vi "STS at various H_MFLI_MF-MD_K3636B_PK_V4.0_withaveraging.vi"() -> ()   [LabVIEW 2016]
uses:
  <instrlib>/Zurich Instruments LabOne/Public/Data/ziTypeDemodSampleSingle.ctl
  <instrlib>/Keithley 2600 Series/Public/Configure/Source/Configure Source (Limit).vi
  <instrlib>/Keithley 2600 Series/Public/Configure/Source/Configure Source (Range).vi
  <instrlib>/Zurich Instruments LabOne/Public/Configure/ziGetValueDemodSampleEx.vi
  <instrlib>/Zurich Instruments LabOne/Zurich Instruments LabOne.lvlib
  <instrlib>/Keithley 2600 Series/Keithley 2600 Series.lvlib
panel:
  in  "DC Current Limit (A)":dbl format="%#_13g"
  in  "Keithley 2636B (channelA)":refnum<visa-resource-name>
  in  "Field ramp rate (T/min)":string="0.05"
  in  "Step 2":dbl[](array[numeric])=[0.005] min=-3000.0 max=3000.0 format="%.1e"
  in  "To 2":dbl[](array[numeric])=[-5.0] min=-3000.0 max=3000.0 format="%.1e"
  in  "From 2":dbl[](array[numeric])=[5.0] min=-3000.0 max=3000.0 format="%.1e"
  in  "Magnet IP Address":string="169.254.46.132"
  in  "Magnetic field stabilization time (s)":dbl=200.0 format="%#_13g"
  out "Magnetic Field (T)":dbl format="%#_13g"
  in  "DC Voltage averaging":dbl=10.0 format="%#_13g"
  out "Demod Sample Out 2":T1={"Timestamps (ticks)"=34359738372, "X (Vrms)"=8.366245757779461e-285, "Y (Vrms)"=1.0096057436928657e-284, "Osc Phase (deg)"=1.69759663376e-313, "Freq (Hz)"=2.607691286315397e-191, "DIO"=4, "AuxIn0 (V)"=0.0, "AuxIn1 (V)"=1.6954746369817e-311, "Trigger"=16}
  out "Demod Sample Out":T1={"Timestamps (ticks)"=34359738372, "X (Vrms)"=8.366245757779461e-285, "Y (Vrms)"=1.0096057436928657e-284, "Osc Phase (deg)"=1.69759663376e-313, "Freq (Hz)"=2.607691286315397e-191, "DIO"=4, "AuxIn0 (V)"=0.0, "AuxIn1 (V)"=1.6954746369817e-311, "Trigger"=16}
  out "Vset (V)":dbl
  in  "stop":bool
  out "Time(s)":dbl
  in  "Delay (s)":dbl=12.0
  out "dI/dV (S)":dbl
  out "dV (V)":dbl
  out "dI (A)":dbl
  in  "MFLI Address":string="DEV4382"
  out "DC Voltage (V)":dbl
  in  "Folder":path=path "D:/Yaojia/KV3Sb5_JJ_004/21-05-2020"
  out "dI/dV vs Voltage":cluster{dbl, "Field Reading":dbl}[](graph)=[{0.0, "Field Reading"=0.0}, {0.0293132694, "Field Reading"=0.0001}, {-0.00546459921, "Field Reading"=0.0002}, {0.0161308434, "Field Reading"=0.00030000000000000003}, {0.0223832692, "Field Reading"=0.0004}, {0.0328436404, "Field Reading"=0.0005}, {0.038420414, "Field Reading"=0.0006000000000000001}, {0.0417674657, "Field Reading"=0.0007000000000000001}, {0.0438858754, "Field Reading"=0.0008000000000000001}, {0.0446854721, "Field Reading"=0.0009000000000000002}, {0.044680018, "Field Reading"=0.001}, {0.0438771516, "Field Reading"=0.0009}, {0.0430695093, "Field Reading"=0.0007999999999999999}, {0.0423949057, "Field Reading"=0.0006999999999999999}, {0.0424006302, "Field Reading"=0.0005999999999999998}, {0.0430089846, "Field Reading"=0.0004999999999999998}, {0.0431435269, "Field Reading"=0.0003999999999999998}, {0.0431290947, "Field Reading"=0.0002999999999999998}, {0.0703335255, "Field Reading"=0.00019999999999999982}, {0.0575145557, "Field Reading"=9.999999999999982e-05}, {0.11367481, "Field Reading"=-1.8973538018496328e-19}, {0.109008679, "Field Reading"=-0.0001000000000000002}, {0.0119374597, "Field Reading"=-0.0002000000000000002}, {-0.0231964252, "Field Reading"=-0.0003000000000000002}, {-0.0302370322, "Field Reading"=-0.0004000000000000002}, {-0.0435009579, "Field Reading"=-0.0005000000000000002}, {-0.0500857587, "Field Reading"=-0.0006000000000000003}, {-0.0527825661, "Field Reading"=-0.0007000000000000003}, {-0.0535569139, "Field Reading"=-0.0008000000000000004}, {-0.0533778669, "Field Reading"=-0.0009000000000000004}, {-0.0526966423, "Field Reading"=-0.001}, {-0.0518844802, "Field Reading"=-0.0009}, {-0.051037725, "Field Reading"=-0.0007999999999999999}, {-0.0502346264, "Field Reading"=-0.0006999999999999999}, {-0.0495006625, "Field Reading"=-0.0005999999999999998}, {-0.0488631228, "Field Reading"=-0.0004999999999999998}, {-0.0482498135, "Field Reading"=-0.0003999999999999998}, {-0.0476401668, "Field Reading"=-0.0002999999999999998}, {-0.0812013466, "Field Reading"=-0.00019999999999999982}, {-0.0619737297, "Field Reading"=-9.999999999999982e-05}]
  out "data":dbl[](array[numeric])=[-0.0619737297, -9.999999999999982e-05, 619.7372970000011]
  in  "Nanovoltmeter 2182a VISA":refnum<visa-resource-name>="GPIB0::7::INSTR"
  in  "Step":dbl[](array[numeric])=[0.005] min=-3000.0 max=3000.0 format="%.1e"
  in  "To":dbl[](array[numeric])=[-5.0] min=-3000.0 max=3000.0 format="%.1e"
  in  "From":dbl[](array[numeric])=[5.0] min=-3000.0 max=3000.0 format="%.1e"
  in  "file name":string="001_STS_m68_57_ac10nA_6.8uV_0.6mK"
  out "File path":path=path "D:/Data/Elena/001_IV_test_RT.dat"
  # ".dat"
  # "Set Voltage (V)"
  # "Set Magnetic Field (T)"
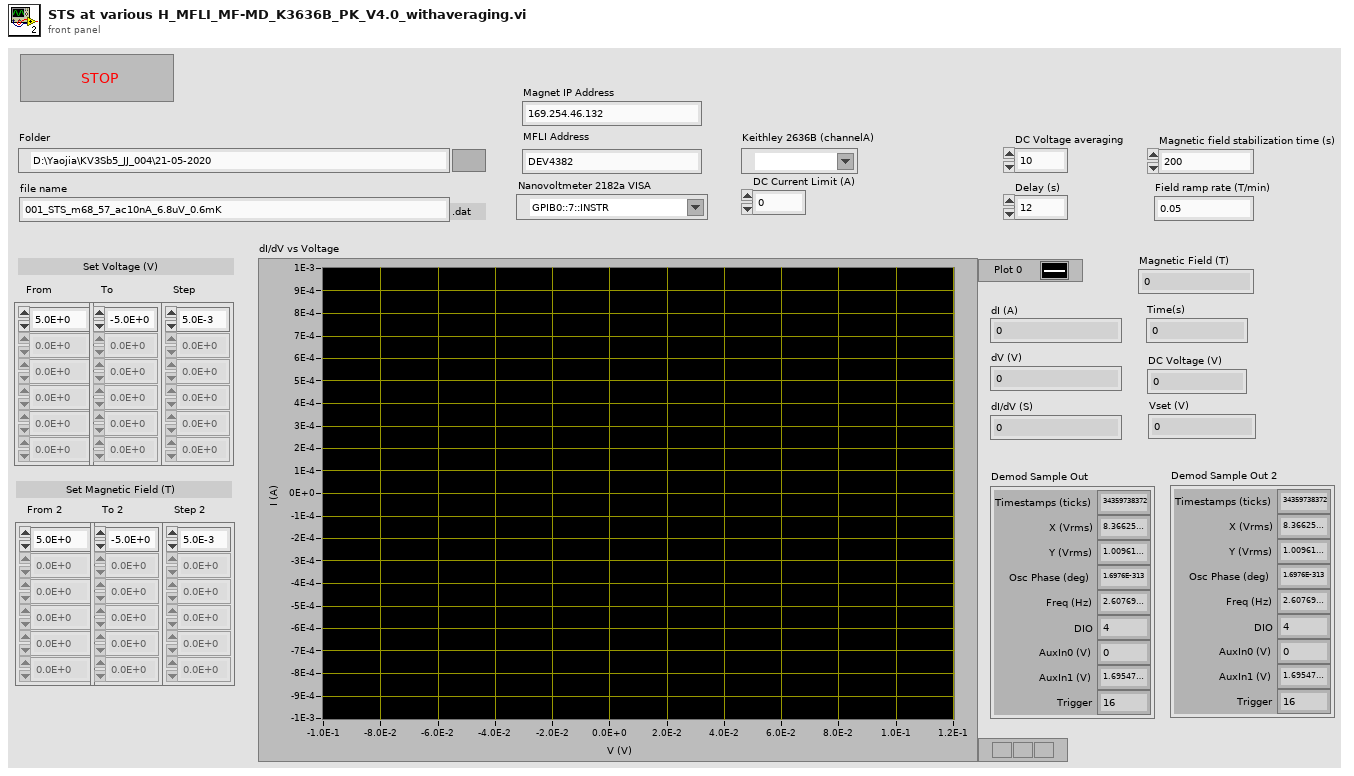
[diagram p1: front panel]
types:
  T1 = typedef "Zurich Instruments LabOne.lvlib/ziTypeDemodSampleSingle.ctl" = cluster{"Timestamps (ticks)":u64, "X (Vrms)":dbl, "Y (Vrms)":dbl, "Osc Phase (deg)":dbl, "Freq (Hz)":dbl, "DIO":u32, "AuxIn0 (V)":dbl, "AuxIn1 (V)":dbl, "Trigger":u32}
  T2 = enum16{"open", "replace", "create", "open or create", "replace or create", "replace or create with confirmation"}
  T3 = typedef "Zurich Instruments LabOne.lvlib/ziTypeHandle.ctl" = cluster{"handleValid":bool, "Conn":u64, "Path Prefix":string, "Handle":u64, "Connected":bool, "Clockbase(s)":dbl}
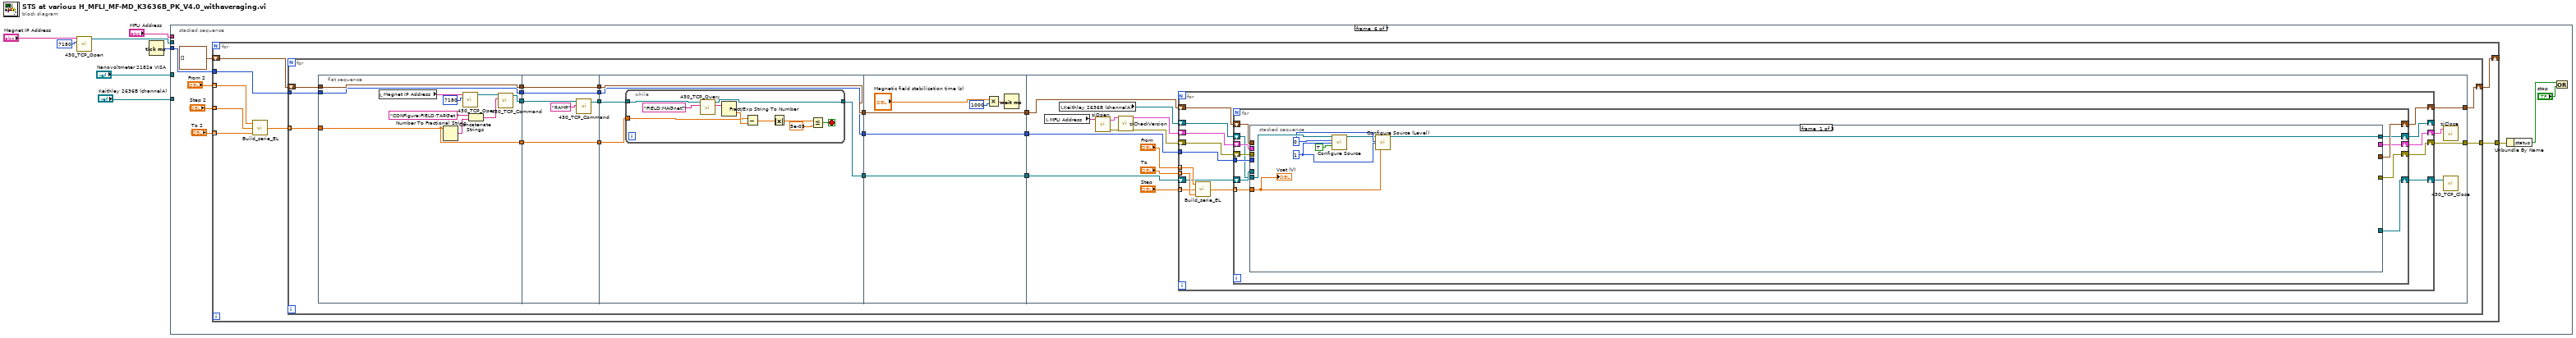
[diagram p0: block diagram]
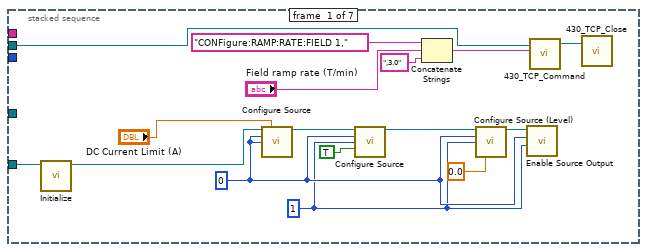
[diagram p2: hidden frame]
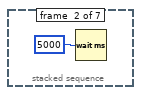
[diagram p3: hidden frame]
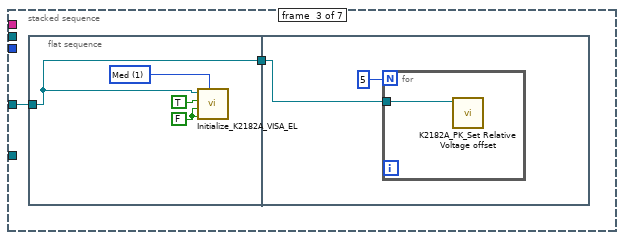
[diagram p4: hidden frame]
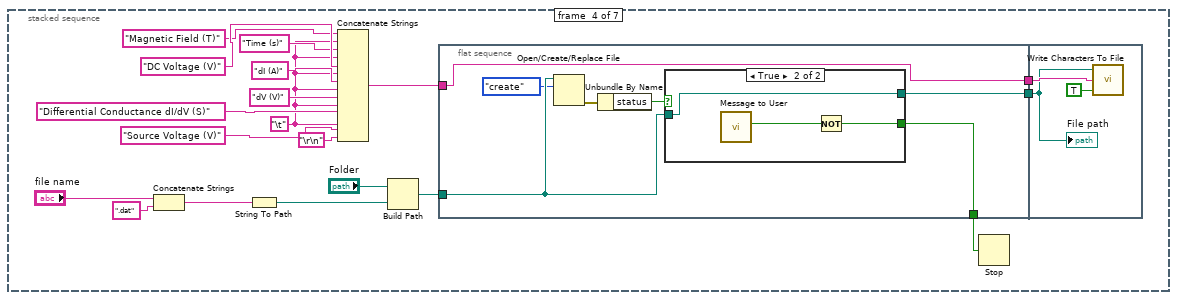
[diagram p5: hidden frame]
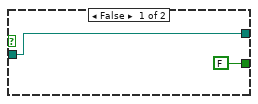
[diagram p6: hidden frame]
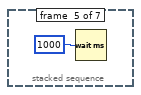
[diagram p7: hidden frame]
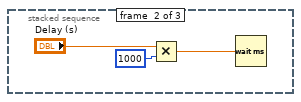
[diagram p8: hidden frame]
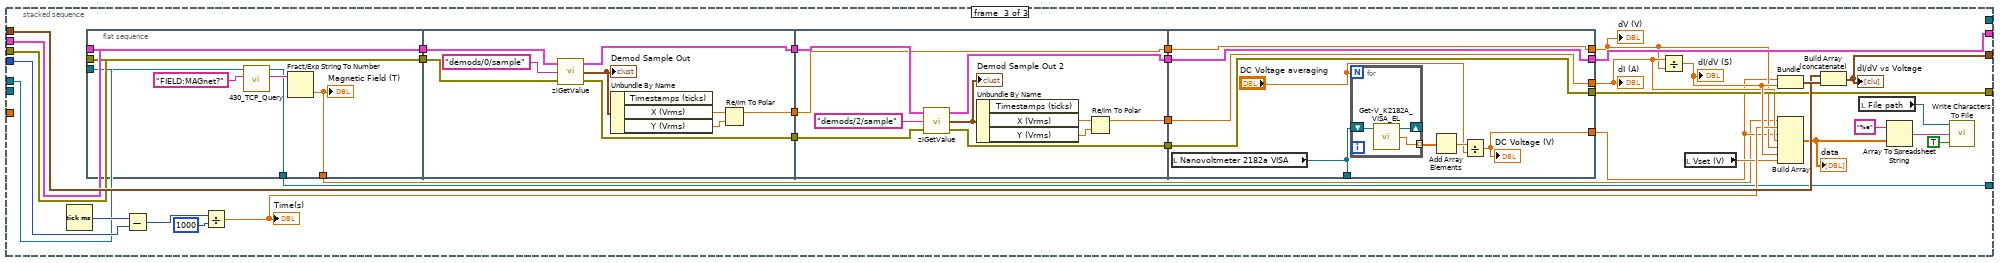
[diagram p9: hidden frame]
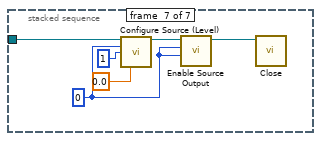
[diagram p10: hidden frame]
diagram:
  n1 = call "430_TCP_Open.vi"("IP Address"="Magnet IP Address", "TCP Port"=7180) -> ("connection ID"=w2:refnum<k5>)  [unwired: 4 in, 2 out]
  n2 = Tick Count (ms)() -> (millisecond timer value=w5:u32)
  n3 = stacked-sequence {
    tunnel: "Nanovoltmeter 2182a VISA" -> [_ _ w26 _ _ _ _]
    tunnel: "MFLI Address" -> [_ _ _ _ _ _ _]
    tunnel: w5 -> [_ _ _ _ _ w75 _]
    tunnel: w2 -> [w18 _ _ _ _ _ _]
    tunnel: "Keithley 2636B (channelA)" -> [w17 _ _ _ _ _ w268]
    frame #0 {
      w11 = 0
      w8 = 1
      n4 = call <instrlib>:"Initialize.vi"("VISA resource name"=w17) -> ("VISA resource name out"=w16:refnum<visa-resource-name>)  [unwired: 9 in, 1 out]
      n5 = call-poly <instrlib>:"Configure Source.vi"("VISA resource name"=w16, "Current Limit (0.1 A)"="DC Current Limit (A)", "Source Measure Unit Channel (0: Channel A)"=w11, "Limit Type (1: Voltage)"=w11) -> ("VISA resource name out"=w15:refnum<visa-resource-name>)  [unwired: 10 in, 1 out]
      n6 = call-poly <instrlib>:"Configure Source.vi"("VISA resource name"=w15, "Source Measure Unit Channel (0: Channel A)"=w11, "Range Type (1: Voltage)"=w8, "Auto Range (T: Enable)"=TRUE) -> ("VISA resource name out"=w14:refnum<visa-resource-name>)  [unwired: 10 in, 1 out]
      n7 = Concatenate Strings("CONFigure:RAMP:RATE:FIELD 1," ("String"), "Field ramp rate (T/min)", ",3.0") -> (w19:string)
      n8 = call <instrlib>:"Configure Source (Level).vi"("VISA resource name"=w14, "Source Measure Unit Channel (0: Channel A)"=w11, "Level Type (1: Voltage)"=w8, "Voltage Level (0 V)"=0.0) -> ("VISA resource name out"=w13:refnum<visa-resource-name>)  [unwired: 10 in, 1 out]
      n9 = call <instrlib>:"Enable Source Output.vi"("Output Mode (0: Turn off)"=w8, "Source Measure Unit Channel (0: Channel A)"=w11, "VISA resource name"=w13) -> ()  [unwired: 7 in, 2 out]
      n10 = call "430_TCP_Command.vi"("Command"=w19, "connection ID"=w18) -> ("connection ID out"=w23:refnum<k5>)  [unwired: 2 in, 2 out]
      n11 = call "430_TCP_Close.vi"("connection ID"=w23) -> ()  [unwired: 1 in, 2 out]
    }
    frame #1 {
      n12 = Wait (ms)(milliseconds to wait=5000) -> ()  [unwired: 1 out]
    }
    frame #2 {
      n13 = flat-sequence {
        tunnel: w26 -> [w27]
        tunnel: [w27] -> w25
        tunnel: w25 -> [w31]
        frame #0 {
          w29 = u16 1 items=["Slow", "Med", "Fast"] ("Rate (NPLC)")
          w30 = FALSE ("Auto range?")
          n14 = call "Initialize_K2182A_VISA_EL.vi"("VISA address"=w27, "Auto range?"=TRUE, "Analog LPass\nFilter?"=w30, "DC\nFilter?"=w30, "Rate (NPLC)"=w29) -> ()  [unwired: 2 in]
        }
        frame #1 {
          n15 = for {
            N: 5 ("Numeric") -> [_]
            tunnel: w31 -> [w33]
            n16 = call "K2182A_PK_Set Relative Voltage offset.vi"("VISA address"=w33) -> ()  [unwired: 11 in]
          }
        }
      }
    }
    frame #3 {
      w35 = "\t"
      n17 = Concatenate Strings("file name", ".dat" ("string")) -> (w49:string)
      n18 = String To Path(string=w49) -> (path=w41:path)
      n19 = Concatenate Strings("Magnetic Field (T)", w35, "Time (s)", w35, "DC Voltage (V)" ("string"), w35, "dI (A)" ("string"), w35, "dV (V)" ("string"), w35, "Differential Conductance dI/dV (S)", w35, "Source Voltage (V)", "\r\n") -> (w50:string)
      n20 = Build Path(base path="Folder", name or relative path=w41) -> (appended path=w40:path)
      n21 = flat-sequence {
        tunnel: w40 -> [w56]
        tunnel: w50 -> [w59]
        tunnel: [w59] -> w52
        tunnel: [w58] -> w47
        tunnel: [w57] -> w51
        tunnel: w52 -> [w66]
        tunnel: w51 -> [w65]
        frame #0 {
          n22 = Open/Create/Replace File(file path (use dialog)=w56, operation (0:open)=T2."create") -> (error out=w55:errorcluster)  [unwired: 4 in, 2 out]
          n23 = Unbundle By Name(w55) -> ("status"=w53:bool)
          n24 = case shown="True" w53 {
            tunnel: [FALSE ("Yes") w63] -> w58
            tunnel: [w60 w62] -> w57
            tunnel: w56 -> [w60 w62]
            frame False {
            }
            frame True {
              n25 = call "Message to User"() -> ("Yes"=w64:bool)  [unwired: 10 in, 1 out]
              n26 = Not(x=w64) -> (.not. x?=w63:bool)
            }
          }
        }
        frame #1 {
          n27 = call <vilib>:"Write Characters To File.vi"("append to file? (new file:F)"=TRUE, "character string"=w66, "file path (dialog if empty)"=w65) -> ()  [unwired: 2 in, 1 out]
          "File path" <- w65
        }
      }
      n28 = Stop(stop? (T)=w47) -> ()
    }
    frame #4 {
      n29 = Wait (ms)(milliseconds to wait=u32 1000) -> ()  [unwired: 1 out]
    }
    frame #5 {
      n30 = for {
        tunnel: w75 -> [w83]
        tunnel: "From 2" -> [w82] mode=indexing
        tunnel: "Step 2" -> [w81] mode=indexing
        tunnel: "To 2" -> [w80] mode=indexing
        shift-right: [w79] -> _
        shift-left: cluster{dbl, "Field Reading":dbl}[] [] -> [w84]
        tunnel: [w77] -> w70
        n31 = call "Build_serie_EL.vi"("end value"=w80, "increment"=w81, "start value"=w82) -> ("output array"=w78:dbl[])
        n32 = for {
          tunnel: w83 -> [w94]
          shift-right: [w93] -> w79
          shift-left: w84 -> [w95]
          tunnel: w78 -> [w92] mode=indexing
          tunnel: [w85] -> w77
          n33 = flat-sequence {
            tunnel: w94 -> [w112]
            tunnel: w95 -> [w113]
            tunnel: [w113] -> w103
            tunnel: [w112] -> w102
            tunnel: w92 -> [w104]
            tunnel: [w105] -> w91
            tunnel: [w104] -> w88
            tunnel: [w119] -> w101
            tunnel: [w118] -> w100
            tunnel: w103 -> [w119]
            tunnel: w102 -> [w118]
            tunnel: w91 -> [w116]
            tunnel: [w115] -> w90
            tunnel: [w114] -> w89
            tunnel: w88 -> [w114]
            tunnel: [w124] -> w99
            tunnel: [w123] -> w98
            tunnel: w101 -> [w124]
            tunnel: w100 -> [w123]
            tunnel: w90 -> [w122]
            tunnel: w89 -> [w121]
            tunnel: [w120] -> w86
            tunnel: [w140] -> w97
            tunnel: [w139] -> w96
            tunnel: w99 -> [w140]
            tunnel: w98 -> [w139]
            tunnel: [w135] -> w87
            tunnel: w86 -> [w135]
            tunnel: [w151] -> w85
            tunnel: w97 -> [w153]
            tunnel: w96 -> [w152]
            tunnel: [w150] -> w93
            tunnel: w87 -> [w149]
            frame #0 {
              n34 = local read "Magnet IP Address"() -> (w107:string)
              n35 = Number To Fractional String(number=w104) -> (F-format string=w109:string)  [unwired: 3 in]
              n36 = call "430_TCP_Open.vi"("IP Address"=w107, "TCP Port"=7180) -> ("connection ID"=w106:refnum<k5>)  [unwired: 4 in, 2 out]
              n37 = Concatenate Strings("CONFigure:FIELD:TARGet " ("String"), w109) -> (w111:string)
              n38 = call "430_TCP_Command.vi"("Command"=w111, "connection ID"=w106) -> ("connection ID out"=w105:refnum<k5>)  [unwired: 2 in, 2 out]
            }
            frame #1 {
              n39 = call "430_TCP_Command.vi"("Command"="RAMP", "connection ID"=w116) -> ("connection ID out"=w115:refnum<k5>)  [unwired: 2 in, 2 out]
            }
            frame #2 {
              n40 = while {
                tunnel: w122 -> [w134]
                tunnel: w121 -> [w129]
                tunnel: [w125] -> w120
                stop <- w127 stop-if-true
                n41 = call "430_TCP_Query.vi"("Command"="FIELD:MAGnet?" ("String"), "connection ID"=w134) -> ("Response"=w133:string, "connection ID out"=w125:refnum<k5>)  [unwired: 5 in, 3 out]
                n42 = Fract/Exp String To Number(string=w133) -> (number=w130:dbl)  [unwired: 3 in, 1 out]
                n43 = Subtract(x=w129, y=w130) -> (x-y=w132:dbl)
                n44 = Absolute Value(x=w132) -> (abs(x)=w131:dbl)
                n45 = Less Or Equal?(x=w131, y=5e-05) -> (x <= y?=w127:bool)
              }
            }
            frame #3 {
              n46 = Multiply(x="Magnetic field stabilization time (s)", y=1000) -> (x*y=w137:dbl)
              n47 = Wait (ms)(milliseconds to wait=w137) -> ()  [unwired: 1 out]
            }
            frame #4 {
              n48 = local read "MFLI Address"() -> (w146:string)
              n49 = local read "Keithley 2636B (channelA)"() -> (w141:refnum<visa-resource-name>)
              n50 = call <instrlib>:"ziOpen.vi"("Address"=w146) -> ("Error Out"=w145:errorcluster, "HandleOut"=w148:T3)  [unwired: 3 in, 1 out]
              n51 = call <instrlib>:"ziCheckVersion.vi"("Handle In"=w148, "Error In"=w145) -> ("Handle Out"=w147:T3, "Error Out"=w144:errorcluster)  [unwired: 11 in, 1 out]
              n52 = for {
                tunnel: "From" -> [w168] mode=indexing
                tunnel: "To" -> [w167] mode=indexing
                tunnel: "Step" -> [w166] mode=indexing
                shift-right: [w170] -> w150
                shift-left: w153 -> [w171]
                tunnel: w152 -> [w165]
                shift-right: [w163] -> w143
                shift-left: w147 -> [w164]
                shift-right: [w162] -> w151
                shift-left: w144 -> [w161]
                shift-right: [w159] -> w142
                shift-left: w149 -> [w160]
                shift-right: [w157] -> _
                shift-left: w141 -> [w158]
                n53 = call "Build_serie_EL.vi"("end value"=w167, "increment"=w166, "start value"=w168) -> ("output array"=w169:dbl[])
                n54 = for {
                  tunnel: w169 -> [w183] mode=indexing
                  shift-right: [w181] -> w170
                  shift-left: w171 -> [w182]
                  tunnel: w165 -> [w180]
                  shift-right: [w178] -> w163
                  shift-left: w164 -> [w179]
                  shift-right: [w177] -> w162
                  shift-left: w161 -> [w176]
                  shift-right: [w174] -> w159
                  shift-left: w160 -> [w175]
                  shift-right: [w172] -> w157
                  shift-left: w158 -> [w173]
                  n55 = stacked-sequence {
                    tunnel: w182 -> [_ _ w226]
                    tunnel: w183 -> [w190 _ _]
                    tunnel: [_ _ w225] -> w181
                    tunnel: w180 -> [_ _ w222]
                    tunnel: w179 -> [_ _ w218]
                    tunnel: [_ _ w217] -> w178
                    tunnel: [_ _ w216] -> w177
                    tunnel: w176 -> [_ _ w215]
                    tunnel: w175 -> [_ _ w196]
                    tunnel: [_ _ w195] -> w174
                    tunnel: w173 -> [w188 _ _]
                    tunnel: [w189 _ _] -> w172
                    frame #0 {
                      w187 = 0
                      w186 = 1
                      n56 = call-poly <instrlib>:"Configure Source.vi"("VISA resource name"=w188, "Source Measure Unit Channel (0: Channel A)"=w187, "Range Type (1: Voltage)"=w186, "Auto Range (T: Enable)"=TRUE) -> ("VISA resource name out"=w184:refnum<visa-resource-name>)  [unwired: 10 in, 1 out]
                      n57 = call <instrlib>:"Configure Source (Level).vi"("VISA resource name"=w184, "Source Measure Unit Channel (0: Channel A)"=w187, "Level Type (1: Voltage)"=w186, "Voltage Level (0 V)"=w190) -> ("VISA resource name out"=w189:refnum<visa-resource-name>)  [unwired: 10 in, 1 out]
                      "Vset (V)" <- w190
                    }
                    frame #1 {
                      n58 = Multiply(x="Delay (s)", y=1000) -> (x*y=w192:dbl)
                      n59 = Wait (ms)(milliseconds to wait=w192) -> ()  [unwired: 1 out]
                    }
                    frame #2 {
                      n60 = Tick Count (ms)() -> (millisecond timer value=w223:u32)
                      n61 = flat-sequence {
                        tunnel: w215 -> [w233]
                        tunnel: w218 -> [w234]
                        tunnel: [w234] -> w198
                        tunnel: [w233] -> w197
                        tunnel: w196 -> [w230]
                        tunnel: [w229] -> w195
                        tunnel: [w228] -> w194
                        tunnel: [w237] -> w208
                        tunnel: [w236] -> w207
                        tunnel: [w235] -> w206
                        tunnel: w198 -> [w239]
                        tunnel: w197 -> [w238]
                        tunnel: w208 -> [w249]
                        tunnel: w207 -> [w248]
                        tunnel: w206 -> [w244]
                        tunnel: [w247] -> w203
                        tunnel: [w246] -> w202
                        tunnel: [w245] -> w201
                        tunnel: [w244] -> w200
                        tunnel: [w259] -> w204
                        tunnel: [w260] -> w205
                        tunnel: [w261] -> w216
                        tunnel: [w262] -> w217
                        tunnel: w203 -> [w262]
                        tunnel: w202 -> [w261]
                        tunnel: w201 -> [w260]
                        tunnel: w200 -> [w259]
                        tunnel: [w256] -> w199
                        tunnel: [w254] -> _
                        frame #0 {
                          n62 = call "430_TCP_Query.vi"("Command"="FIELD:MAGnet?" ("String"), "connection ID"=w230) -> ("Response"=w232:string, "connection ID out"=w229:refnum<k5>)  [unwired: 5 in, 3 out]
                          n63 = Fract/Exp String To Number(string=w232) -> (number=w228:dbl)  [unwired: 3 in, 1 out]
                          "Magnetic Field (T)" <- w228
                        }
                        frame #1 {
                          n64 = call-poly <instrlib>:"ziGetValue.vi"("error in"=w238, "Path"="demods/0/sample", "Handle In"=w239) -> ("error out"=w236:errorcluster, "Demod Sample Out"=w242:T1, "Handle Out"=w237:T3)
                          "Demod Sample Out" <- w242
                          n65 = Unbundle By Name(w242) -> ("X (Vrms)"=w241:dbl, "Y (Vrms)"=w240:dbl)  [unwired: 1 out]
                          n66 = Re/Im To Polar(2:w240, 3:w241) -> (1:w235:dbl)  [unwired: 1 out]
                        }
                        frame #2 {
                          n67 = call-poly <instrlib>:"ziGetValue.vi"("error in"=w248, "Path"="demods/2/sample", "Handle In"=w249) -> ("error out"=w246:errorcluster, "Demod Sample Out"=w252:T1, "Handle Out"=w247:T3)
                          "Demod Sample Out 2" <- w252
                          n68 = Unbundle By Name(w252) -> ("X (Vrms)"=w251:dbl, "Y (Vrms)"=w250:dbl)  [unwired: 1 out]
                          n69 = Re/Im To Polar(2:w250, 3:w251) -> (1:w245:dbl)  [unwired: 1 out]
                        }
                        frame #3 {
                          n70 = local read "Nanovoltmeter 2182a VISA"() -> (w254:refnum<visa-resource-name>)
                          n71 = for {
                            N: "DC Voltage averaging" -> [_]
                            tunnel: [w264] -> w257 mode=indexing
                            shift-right: [w263] -> _
                            shift-left: w254 -> [w265]
                            n72 = call "Get-V_K2182A_VISA_EL.vi"("VISA K2182A"=w265) -> ("V (V)"=w264:dbl, "VISA K2182A"=w263:refnum<visa-resource-name>)  [unwired: 2 in, 1 out]
                          }
                          n73 = Add Array Elements(numeric array=w257) -> (sum=w258:dbl)
                          n74 = Divide(x=w258, y="DC Voltage averaging") -> (x/y=w256:dbl)
                          "DC Voltage (V)" <- w256
                        }
                      }
                      n75 = Subtract(x=w223, y=w222) -> (x-y=w221:u32)
                      n76 = Divide(x=w221, y=1000) -> (x/y=w219:dbl)
                      "Time(s)" <- w219
                      n77 = Divide(x=w205, y=w204) -> (x/y=w224:dbl)
                      "dI/dV (S)" <- w224
                      n78 = local read "Vset (V)"() -> (w209:dbl)
                      n79 = Bundle(w199, w224) -> (w227:cluster{dbl, dbl})  [unwired: 1 in]
                      n80 = Build Array(w194, w219, w199, w205, w204, w224, w209) -> (w210:dbl[])
                      "data" <- w210
                      n81 = Build Array (concatenate)(w226, w227) -> (w225:cluster{dbl, "Field Reading":dbl}[])
                      "dI/dV vs Voltage" <- w225
                      n82 = local read "File path"() -> (w212:path)
                      n83 = Array To Spreadsheet String(array=w210, 3:"%e" ("format string")) -> (spreadsheet string=w213:string)  [unwired: 1 in]
                      n84 = call <vilib>:"Write Characters To File.vi"("append to file? (new file:F)"=TRUE, "character string"=w213, "file path (dialog if empty)"=w212) -> ()  [unwired: 2 in, 1 out]
                      "dI (A)" <- w205
                      "dV (V)" <- w204
                    }
                  }
                }
              }
              n85 = call <instrlib>:"ziClose.vi"("Handle In"=w143) -> ()  [unwired: 1 in, 4 out]
              n86 = call "430_TCP_Close.vi"("connection ID"=w142) -> ()  [unwired: 1 in, 2 out]
            }
          }
        }
      }
      n87 = Unbundle By Name(w70) -> ("status"=w69:bool)
      n88 = Or(x=w69, y="stop") -> ()  [unwired: 1 out]
    }
    frame #6 {
      w267 = 0
      n89 = call <instrlib>:"Configure Source (Level).vi"("VISA resource name"=w268, "Source Measure Unit Channel (0: Channel A)"=w267, "Level Type (1: Voltage)"=1, "Voltage Level (0 V)"=0.0) -> ("VISA resource name out"=w271:refnum<visa-resource-name>)  [unwired: 10 in, 1 out]
      n90 = call <instrlib>:"Enable Source Output.vi"("Output Mode (0: Turn off)"=w267, "Source Measure Unit Channel (0: Channel A)"=w267, "VISA resource name"=w271) -> ("VISA resource name out"=w266:refnum<visa-resource-name>)  [unwired: 7 in, 1 out]
      n91 = call <instrlib>:"Close.vi"("VISA resource name"=w266) -> ()  [unwired: 10 in, 1 out]
    }
  }
